vi "Video livestream 1Hz (TCP SERVER).vi"(1 "TCP/IP port":u16=80, 2 "VideoMode":u32, 3 "Interface name":T1="Travcam") -> (0 "Error Out":errorcluster)   [LabVIEW 2015]
doc: "This VI must be loaded when the camera server starts, and also in the list of exported VIs. This VI is not to run directly."
uses:
  <vilib>/userdefined/High Color/IMAQdx.ctl
  <vilib>/vision/driver/IMAQdx.llb/IMAQdx Camera Control Mode.ctl
  <vilib>/vision/driver/NI_Vision_Acquisition_Software.lvlib
  <resource>/objmgr/imaqdx.rc
panel:
  in  "Stop":bool
  out "Snapshot":T2(plugin-control)
  # "PN 27/08/2015"
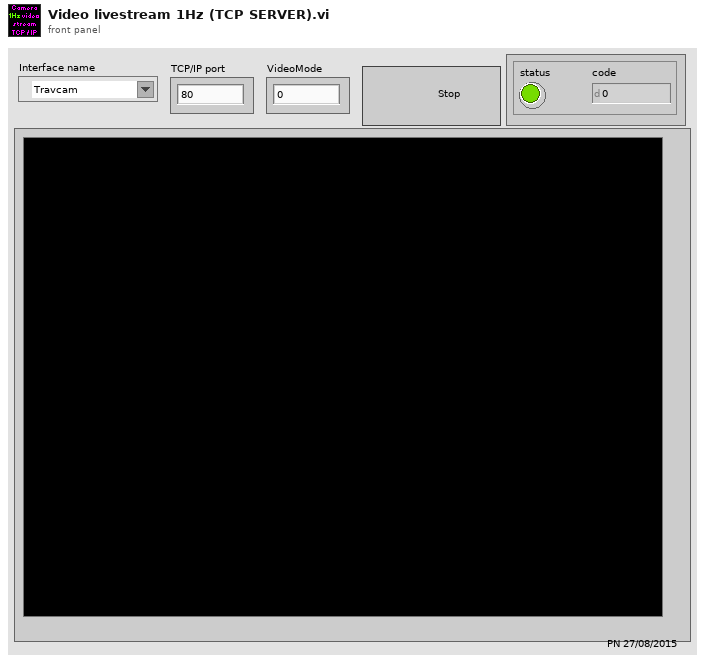
[diagram p1: front panel]
types:
  T1 = typedef "IMAQdx.ctl" = refnum<k21>
  T2 = typedef "IMAQ Image.ctl" = refnum<image>
  T3 = typedef "Image Type" = u32
  T4 = typedef "NI_Vision_Acquisition_Software.lvlib/IMAQdx Camera Control Mode.ctl" = enum32{"Controller", "Listener"}
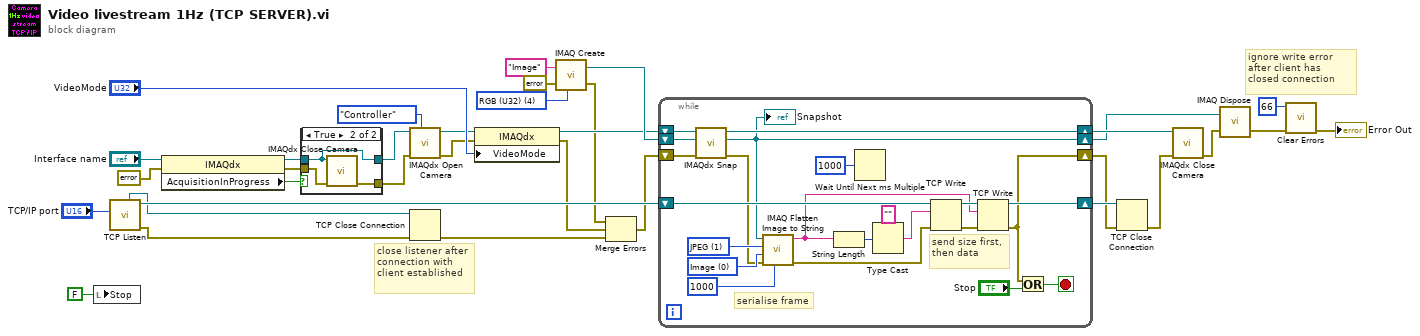
[diagram p0: block diagram]
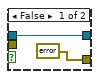
[diagram p2: hidden frame]
diagram:
  w29 = T3 4 items=["Grayscale (U8)", "Grayscale (I16)", "Grayscale (SGL)", "Complex (CSG)", "RGB (U32)", "HSL (U32)", "RGB (U64)", "Grayscale (U16)"] ("Image Type")
  # "ignore write error after client has closed connection"
  # "close listener after connection with client established"
  n1 = local write "Stop"(FALSE ("Stop")) -> ()
  n2 = call <vilib>:"TCP Listen.vi"("port"="TCP/IP port") -> ("error out"=w16:errorcluster, "connection ID"=w33:refnum<k5>, "listener ID"=w17:refnum<k5>)  [unwired: 6 in, 2 out]
  n3 = property class="IMAQdx"(reference="Interface name", error in=errorcluster {"status"=FALSE, "code"=0, "source"=""}) -> (reference out=w5:T1, error out=w3:errorcluster, "AcquisitionInProgress"=w2:bool)
  n4 = case shown="True" w2 {
    tunnel: w5 -> [w36 w37]
    tunnel: w3 -> [_ w39]
    tunnel: [errorcluster {"status"=FALSE, "code"=0, "source"=""} ("error in") w38] -> w1
    tunnel: [w36 w37] -> w4
    frame False {
    }
    frame True {
      n5 = call <vilib>:"IMAQdx Close Camera.vi"("error in"=w39, "Session In"=w37) -> ("error out"=w38:errorcluster)  [unwired: 9 in]
    }
  }
  n6 = call <vilib>:"IMAQdx Open Camera.vi"("Camera Control Mode"=IMAQdx_Camera_Control_Mode."Controller", "error in"=w1, "Session In"=w4) -> ("error out"=w23:errorcluster, "Session Out"=w22:T1)  [unwired: 7 in]
  n7 = TCP Close Connection(connection ID=w17, error in (no error)=w16) -> (error out=w15:errorcluster)  [unwired: 1 in, 1 out]
  n8 = property class="IMAQdx"(reference=w22, error in=w23, "VideoMode"="VideoMode") -> (reference out=w24:T1, error out=w20:errorcluster)
  n9 = call "IMAQ Create"("Image Name"="Image", "Image Type"=w29, "error in (no error)"=errorcluster {"status"=FALSE, "code"=0, "source"=""} ("error in")) -> ("New Image"=w28:T2, "error out"=w8:errorcluster)  [unwired: 2 in]
  n10 = Merge Errors(w8, w20, w15) -> (w19:errorcluster)
  n11 = while {
    shift-right: [w42] -> w27
    shift-left: w24 -> [w46]
    shift-right: [w41] -> w26
    shift-left: w28 -> [w45]
    shift-right: [w48] -> w13
    shift-left: w19 -> [w44]
    shift-right: [w49] -> w18
    shift-left: w33 -> [w54]
    stop <- w61 stop-if-true
    w57 = 1 items=["None", "JPEG", "PACKED BINARY"] ("Compression (None)")
    w58 = 0 items=["Image", "Image and Vision Info", "Reference to Image"] ("Type of Flatten (Image and Vision Info)")
    # "serialise frame"
    # "send size first, then data"
    n12 = call <vilib>:"IMAQdx Snap.vi"("error in"=w44, "Image In"=w45, "Session In"=w46) -> ("error out"=w43:errorcluster, "Image Out"=w41:T2, "Session Out"=w42:T1)  [unwired: 6 in]
    "Snapshot" <- w41
    n13 = call "IMAQ Flatten Image to String"("Quality (750)"=1000, "error in (no error)"=w43, "Type of Flatten (Image and Vision Info)"=w58, "Compression (None)"=w57, "Image"=w41) -> ("error out"=w52:errorcluster, "Data String"=w47:string)  [unwired: 5 in]
    n14 = String Length(string=w47) -> (length=w56:i32)
    n15 = Wait Until Next ms Multiple(millisecond multiple=u32 1000) -> ()  [unwired: 1 out]
    n16 = Type Cast(type="", x=w56) -> (*(type *) &x=w53:string)
    n17 = TCP Write(connection ID=w54, data in=w53, error in (no error)=w52) -> (connection ID out=w50:refnum<k5>, error out=w51:errorcluster)  [unwired: 1 in, 1 out]
    n18 = TCP Write(connection ID=w50, data in=w47, error in (no error)=w51) -> (connection ID out=w49:refnum<k5>, error out=w48:errorcluster)  [unwired: 1 in, 1 out]
    n19 = Or(x=w48, y="Stop") -> (x .or. y?=w61:bool)
  }
  n20 = TCP Close Connection(connection ID=w18, error in (no error)=w13) -> (error out=w12:errorcluster)  [unwired: 1 in, 1 out]
  n21 = call <vilib>:"IMAQdx Close Camera.vi"("error in"=w12, "Session In"=w27) -> ("error out"=w25:errorcluster)  [unwired: 9 in]
  n22 = call "IMAQ Dispose"("Image"=w26, "error in (no error)"=w25) -> ("error out"=w9:errorcluster)  [unwired: 4 in]
  n23 = call <vilib>:"Clear Errors.vi"("error in (no error)"=w9, "specific error code to clear (0: all)"=66) -> ("error out"=→"Error Out":errorcluster)  [unwired: 4 in, 1 out]
